vi "ReadData6.vi"() -> ()   [LabVIEW 2013]
uses:
  <vilib>/Utility/file.llb/Read From Spreadsheet File (DBL).vi
  <vilib>/Analysis/NI_AALPro.lvlib
  <vilib>/Analysis/NI_AALBase.lvlib
panel:
  out "Residual (V)":dbl=0.00030684756196116164 format="%#_3g"
  in  "1st sweep":i32=400
  in  "# of sweeps":i32=500
  out "Mean Error":dbl=0.0011249589574806795 format="%#_2g"
  out "Mean Area":dbl=0.018285831544207886 format="%#_4g"
  out "Spectrum #":i32=499
  out "Chars":i32=640716
  out "Fcen":dbl=213.0 format="%#_13g"
  in  "Fmin":dbl=212.8 format="%#_13g"
  in  "Fmax":dbl=213.2 format="%#_13g"
  out "# Data points":i32=81
  out "Peak Area (V-MHz)":dbl=0.016394272964669283 format="%#_3g"
  in  "Offset V":dbl=0.118 format="%#_3g"
  out "RMS Fit Error (V)":dbl=0.005928071319865591 format="%#_2g"
  in  "Start sigma (V)":dbl=0.01 format="%#_13g"
  in  "Start offset (V)":dbl format="%#_13g"
  out "FWHM (MHz)":dbl=0.06506841897793307 format="%#_3g"
  out "Center Freq (MHz)":dbl=213.0058317158631
  out "Amplitude (V)":dbl=0.2362707434086921 format="%#_3g"
  out "NMR Graph + Fit":cluster{cluster{dbl, "Numeric":dbl}[]}[](graph)=[{[{212.8, "Numeric"=2.363778842495368e-13}, {212.805, "Numeric"=8.902600611203184e-13}, {212.81, "Numeric"=3.2453766315993214e-12}, {212.815, "Numeric"=1.1451212757939673e-11}, {212.82000000000002, "Numeric"=3.910893842297015e-11}, {212.82500000000002, "Numeric"=1.2928220069997044e-10}, {212.83, "Numeric"=4.136562682898891e-10}, {212.835, "Numeric"=1.2810870705016114e-09}, {212.84, "Numeric"=3.8402177546863156e-09}, {212.845, "Numeric"=1.1142206913060541e-08}, {212.85000000000002, "Numeric"=3.129138254036874e-08}, {212.85500000000002, "Numeric"=8.505825122671001e-08}, {212.86, "Numeric"=2.237929040306476e-07}, {212.865, "Numeric"=5.699205791883683e-07}, {212.87, "Numeric"=1.4048195137059482e-06}, {212.875, "Numeric"=3.3516980604120123e-06}, {212.88, "Numeric"=7.740114936173332e-06}, {212.88500000000002, "Numeric"=1.7300876112483814e-05}, {212.89000000000001, "Numeric"=3.7430613688616755e-05}, {212.895, "Numeric"=7.838337581506647e-05}, {212.9, "Numeric"=0.00015887631007146483}, {212.905, "Numeric"=0.00031169690538213084}, {212.91, "Numeric"=0.0005918940865861797}, {212.915, "Numeric"=0.0010879117729213964}, {212.92000000000002, "Numeric"=0.0019354480411383043}, {212.925, "Numeric"=0.0033327867181186036}, {212.93, "Numeric"=0.005554841759608194}, {212.935, "Numeric"=0.008961362106463306}, {212.94, "Numeric"=0.013993118951798314}, {212.945, "Numeric"=0.021149163288258232}, {212.95, "Numeric"=0.030939266937258292}, {212.955, "Numeric"=0.04380916881708956}, {212.96, "Numeric"=0.06004241781343646}, {212.965, "Numeric"=0.07965068147769151}, {212.97, "Numeric"=0.10227252641250671}, {212.975, "Numeric"=0.12710617145852252}, {212.98, "Numeric"=0.1529017498753417}, {212.985, "Numeric"=0.17803133094838797}, {212.99, "Numeric"=0.2006404930271906}, {212.995, "Numeric"=0.21886630139748287}, {213.0, "Numeric"=0.23108799060021426}, {213.005, "Numeric"=0.23616417532011164}, {213.01, "Numeric"=0.23360859930023833}, {213.015, "Numeric"=0.22366694055030456}, {213.02, "Numeric"=0.20727786843888132}, {213.025, "Numeric"=0.18592690303473344}, {213.03, "Numeric"=0.16142459357518082}, {213.035, "Numeric"=0.13565485226578491}, {213.04, "Numeric"=0.11034156228151969}, {213.045, "Numeric"=0.08687225389622207}, {213.05, "Numeric"=0.06620049167290953}, {213.055, "Numeric"=0.048829188344330414}, {213.06, "Numeric"=0.034860688528937034}, {213.065, "Numeric"=0.0240896550155223}, {213.07, "Numeric"=0.01611251614068875}, {213.075, "Numeric"=0.010431201026979395}, {213.07999999999998, "Numeric"=0.006536472367332196}, {213.085, "Numeric"=0.003964520874143986}, {213.09, "Numeric"=0.002327427454472583}, {213.095, "Numeric"=0.0013225124280330355}, {213.1, "Numeric"=0.0007273803016944781}, {213.105, "Numeric"=0.0003872232932841738}, {213.10999999999999, "Numeric"=0.00019952603746162975}, {213.11499999999998, "Numeric"=9.951208960666663e-05}, {213.12, "Numeric"=4.8038593002941276e-05}, {213.125, "Numeric"=2.244620250801022e-05}, {213.13, "Numeric"=1.0151579953305604e-05}, {213.135, "Numeric"=4.443882496333521e-06}, {213.14, "Numeric"=1.8829104219250282e-06}, {213.14499999999998, "Numeric"=7.722091021339781e-07}, {213.14999999999998, "Numeric"=3.0653377834327045e-07}, {213.155, "Numeric"=1.1777684740226682e-07}, {213.16, "Numeric"=4.380056137615701e-08}, {213.165, "Numeric"=1.5766583426547003e-08}, {213.17, "Numeric"=5.493304516125009e-09}, {213.17499999999998, "Numeric"=1.85254139238475e-09}, {213.17999999999998, "Numeric"=6.047005050400953e-10}, {213.185, "Numeric"=1.9105170025266017e-10}, {213.19, "Numeric"=5.842512463679149e-11}, {213.195, "Numeric"=1.7293645527105895e-11}, {213.2, "Numeric"=4.954634507187724e-12}]}, {[{212.8, "Numeric"=0.004967440902254871}, {212.805, "Numeric"=-0.000296310531098675}, {212.81, "Numeric"=0.0010636834632183044}, {212.815, "Numeric"=0.00015015557407134416}, {212.82000000000002, "Numeric"=-0.003892310112972727}, {212.82500000000002, "Numeric"=-0.0014725852316157077}, {212.83, "Numeric"=-0.0023240371022075646}, {212.835, "Numeric"=-0.0017785572758793513}, {212.84, "Numeric"=-0.0022748424462961697}, {212.845, "Numeric"=7.121507719683851e-05}, {212.85000000000002, "Numeric"=-0.0002230889786892259}, {212.85500000000002, "Numeric"=0.00032456477231700603}, {212.86, "Numeric"=0.0013406520267375912}, {212.865, "Numeric"=0.002099375696453364}, {212.87, "Numeric"=0.0017847176492894966}, {212.875, "Numeric"=0.002550001113168818}, {212.88, "Numeric"=0.004441810296443963}, {212.88500000000002, "Numeric"=0.0011790998212828441}, {212.89000000000001, "Numeric"=0.005336953465366208}, {212.895, "Numeric"=0.005338041130925775}, {212.9, "Numeric"=0.004725033919440696}, {212.905, "Numeric"=0.005706776114412319}, {212.91, "Numeric"=0.006424525086713882}, {212.915, "Numeric"=0.007215254766544911}, {212.92000000000002, "Numeric"=0.004857810252633505}, {212.925, "Numeric"=0.007289539069902403}, {212.93, "Numeric"=0.002345657327556934}, {212.935, "Numeric"=0.004036724358499058}, {212.94, "Numeric"=-0.0006079531606907433}, {212.945, "Numeric"=-0.0028473223096827822}, {212.95, "Numeric"=-0.006544833228898432}, {212.955, "Numeric"=-0.008340857293439667}, {212.96, "Numeric"=-0.007216929546337303}, {212.965, "Numeric"=-0.004868895325288948}, {212.97, "Numeric"=0.003928908530641085}, {212.975, "Numeric"=0.008001653945618654}, {212.98, "Numeric"=0.012537203961757202}, {212.985, "Numeric"=0.01153786978325408}, {212.99, "Numeric"=0.006982401156061391}, {212.995, "Numeric"=0.0028520337900996987}, {213.0, "Numeric"=-0.0014723593376892111}, {213.005, "Numeric"=0.00010656764861838731}, {213.01, "Numeric"=-0.001386202902327774}, {213.015, "Numeric"=0.0048242795597373545}, {213.02, "Numeric"=0.009357326020612403}, {213.025, "Numeric"=0.01427539180160631}, {213.03, "Numeric"=0.01630984322515823}, {213.035, "Numeric"=0.012107750359368095}, {213.04, "Numeric"=0.007440163880240178}, {213.045, "Numeric"=-0.0030114071032364916}, {213.05, "Numeric"=-0.0064734824955001696}, {213.055, "Numeric"=-0.012187842950161915}, {213.06, "Numeric"=-0.01173342947034581}, {213.065, "Numeric"=-0.012007881761045145}, {213.07, "Numeric"=-0.010099588374144507}, {213.075, "Numeric"=-0.007674067897161301}, {213.07999999999998, "Numeric"=-0.008394259719215159}, {213.085, "Numeric"=-0.0052108737863584675}, {213.09, "Numeric"=-0.007589538010539377}, {213.095, "Numeric"=-0.005782368213358102}, {213.1, "Numeric"=-0.006088845641424775}, {213.105, "Numeric"=-0.0056869143330867886}, {213.10999999999999, "Numeric"=-0.00460497224075844}, {213.11499999999998, "Numeric"=-0.004840702366151415}, {213.12, "Numeric"=-0.0023242423109984802}, {213.125, "Numeric"=-0.0046342158474045785}, {213.13, "Numeric"=-0.0028768351709986197}, {213.135, "Numeric"=-0.002149579880285491}, {213.14, "Numeric"=0.00012217112966355715}, {213.14499999999998, "Numeric"=0.0004808905855907135}, {213.14999999999998, "Numeric"=0.0004397852216782692}, {213.155, "Numeric"=0.002021341374489691}, {213.16, "Numeric"=0.00179984490571965}, {213.165, "Numeric"=0.002898880909576887}, {213.17, "Numeric"=0.0015827486301250456}, {213.17499999999998, "Numeric"=0.003769076235776016}, {213.17999999999998, "Numeric"=0.0020295840182770275}, {213.185, "Numeric"=0.0004289023396565735}, {213.19, "Numeric"=0.0002501441304236038}, {213.195, "Numeric"=-0.0020244309700458182}, {213.2, "Numeric"=-0.003536579183989867}]}, {[{212.8, "Numeric"=0.004967440902491249}, {212.805, "Numeric"=-0.0002963105302084149}, {212.81, "Numeric"=0.001063683466463681}, {212.815, "Numeric"=0.00015015558552255691}, {212.82000000000002, "Numeric"=-0.0038923100738637887}, {212.82500000000002, "Numeric"=-0.0014725851023335071}, {212.83, "Numeric"=-0.002324036688551296}, {212.835, "Numeric"=-0.0017785559947922807}, {212.84, "Numeric"=-0.0022748386060784153}, {212.845, "Numeric"=7.122621940375157e-05}, {212.85000000000002, "Numeric"=-0.00022305768730668553}, {212.85500000000002, "Numeric"=0.0003246498305682327}, {212.86, "Numeric"=0.0013408758196416218}, {212.865, "Numeric"=0.002099945617032552}, {212.87, "Numeric"=0.0017861224688032027}, {212.875, "Numeric"=0.00255335281122923}, {212.88, "Numeric"=0.004449550411380137}, {212.88500000000002, "Numeric"=0.0011964006973953277}, {212.89000000000001, "Numeric"=0.0053743840790548255}, {212.895, "Numeric"=0.0054164245067408415}, {212.9, "Numeric"=0.004883910229512162}, {212.905, "Numeric"=0.006018473019794451}, {212.91, "Numeric"=0.007016419173300062}, {212.915, "Numeric"=0.008303166539466307}, {212.92000000000002, "Numeric"=0.00679325829377181}, {212.925, "Numeric"=0.010622325788021006}, {212.93, "Numeric"=0.007900499087165128}, {212.935, "Numeric"=0.012998086464962363}, {212.94, "Numeric"=0.013385165791107571}, {212.945, "Numeric"=0.01830184097857545}, {212.95, "Numeric"=0.02439443370835986}, {212.955, "Numeric"=0.03546831152364989}, {212.96, "Numeric"=0.05282548826709915}, {212.965, "Numeric"=0.07478178615240257}, {212.97, "Numeric"=0.1062014349431478}, {212.975, "Numeric"=0.13510782540414118}, {212.98, "Numeric"=0.1654389538370989}, {212.985, "Numeric"=0.18956920073164205}, {212.99, "Numeric"=0.20762289418325197}, {212.995, "Numeric"=0.22171833518758255}, {213.0, "Numeric"=0.22961563126252504}, {213.005, "Numeric"=0.23627074296873002}, {213.01, "Numeric"=0.23222239639791054}, {213.015, "Numeric"=0.22849122011004191}, {213.02, "Numeric"=0.21663519445949372}, {213.025, "Numeric"=0.20020229483633978}, {213.03, "Numeric"=0.17773443680033904}, {213.035, "Numeric"=0.147762602625153}, {213.04, "Numeric"=0.11778172616175986}, {213.045, "Numeric"=0.08386084679298558}, {213.05, "Numeric"=0.05972700917740937}, {213.055, "Numeric"=0.0366413453941685}, {213.06, "Numeric"=0.023127259058591223}, {213.065, "Numeric"=0.012081773254477155}, {213.07, "Numeric"=0.006012927766544244}, {213.075, "Numeric"=0.002757133129818095}, {213.07999999999998, "Numeric"=-0.0018577873518829636}, {213.085, "Numeric"=-0.0012463529122144813}, {213.09, "Numeric"=-0.005262110556066795}, {213.095, "Numeric"=-0.004459855785325067}, {213.1, "Numeric"=-0.005361465339730297}, {213.105, "Numeric"=-0.005299691039802616}, {213.10999999999999, "Numeric"=-0.00440544620329681}, {213.11499999999998, "Numeric"=-0.004741190276544749}, {213.12, "Numeric"=-0.0022762037179955394}, {213.125, "Numeric"=-0.004611769644896568}, {213.13, "Numeric"=-0.002866683591045314}, {213.135, "Numeric"=-0.002145135997789158}, {213.14, "Numeric"=0.00012405404008548218}, {213.14499999999998, "Numeric"=0.0004816627946928475}, {213.14999999999998, "Numeric"=0.0004400917554566125}, {213.155, "Numeric"=0.0020214591513370932}, {213.16, "Numeric"=0.001799888706281026}, {213.165, "Numeric"=0.0028988966761603133}, {213.17, "Numeric"=0.001582754123429562}, {213.17499999999998, "Numeric"=0.0037690780883174084}, {213.17999999999998, "Numeric"=0.002029584622977533}, {213.185, "Numeric"=0.0004289025307082737}, {213.19, "Numeric"=0.0002501441888487284}, {213.195, "Numeric"=-0.002024430952752173}, {213.2, "Numeric"=-0.0035365791790352326}]}]
  out "File size (bytes)":i32=1284000
  out "File name":string="C:\\Documents and Settings\\Patrick McGaughey\\Desktop\\rssmt\\NMR3489061581.xls"
  # "Gaussian Fit Results"
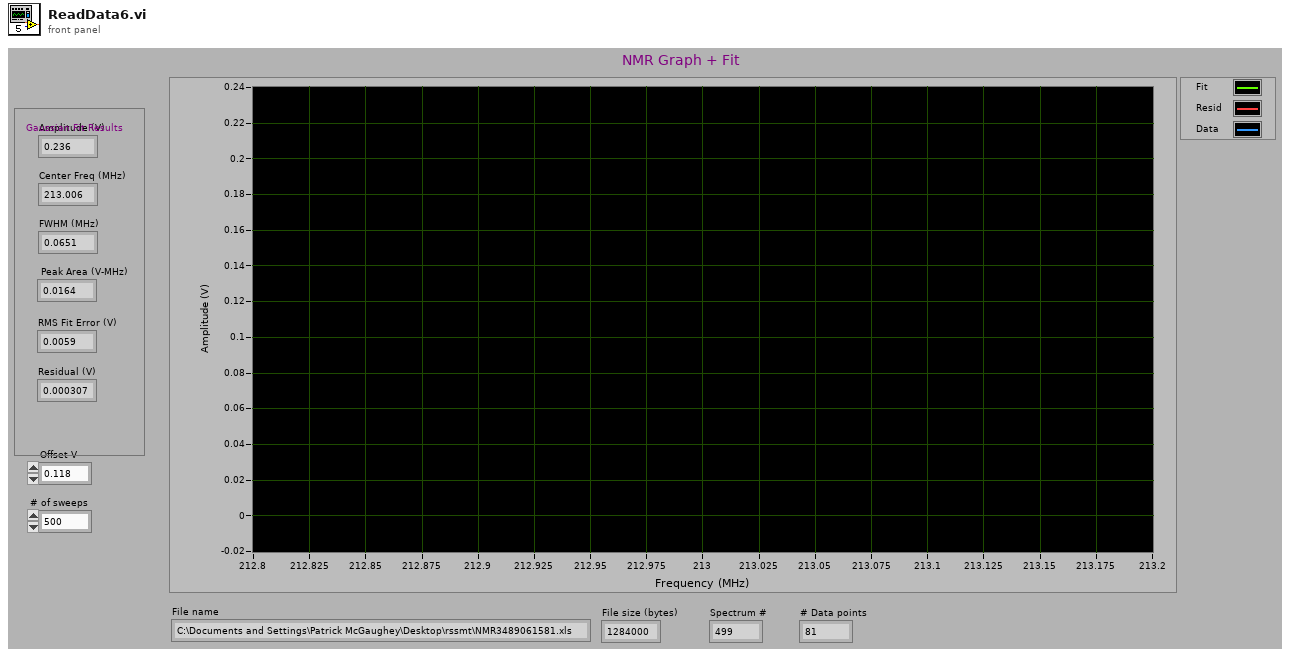
[diagram p1: front panel]
types:
  T1 = cluster{dbl, dbl, "Start sigma (V)":dbl, "Start offset (V)":dbl}
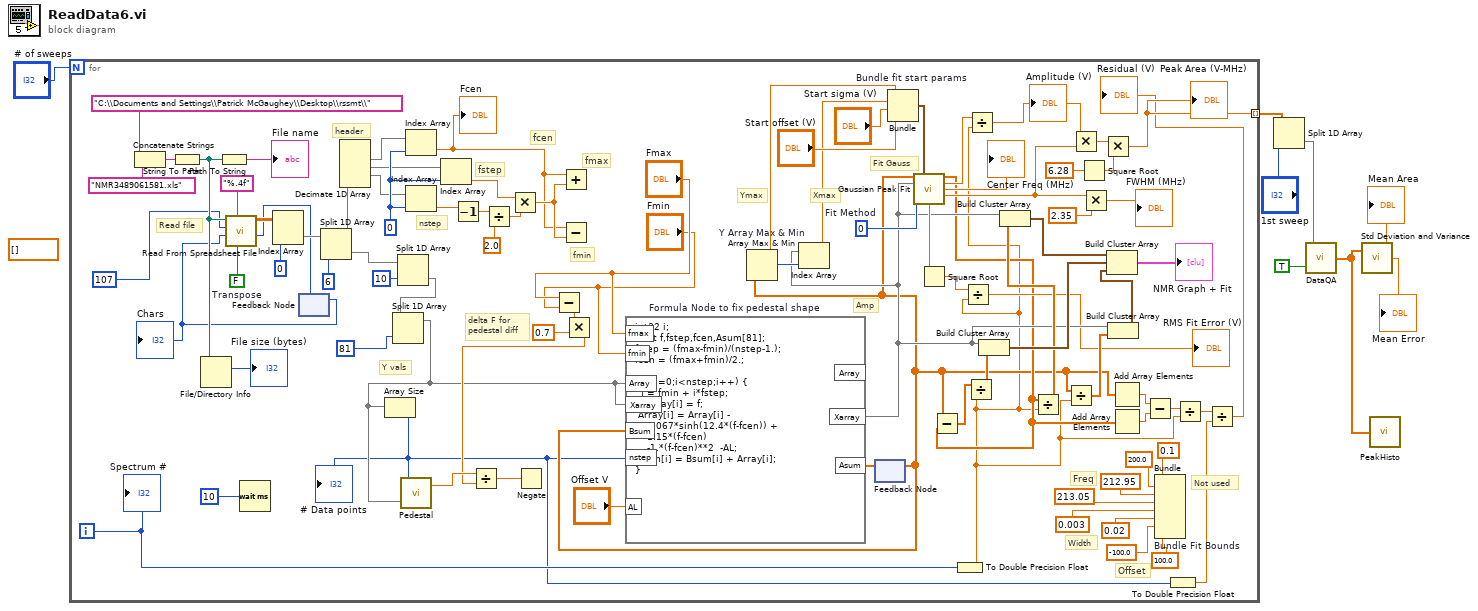
[diagram p0: block diagram]
diagram:
  (unwired) dbl[] []
  n1 = for {
    N: "# of sweeps" -> [_]
    tunnel: [w49] -> w3 mode=indexing
    i -> [w44]
    w60 = 0
    w86 = 0  # Fit Method
    w94 = FALSE  # Transpose
    # "Offset"
    # "Width"
    # "Freq"
    # "Not used"
    # "Fit Gauss"
    # "Read file"
    # "header"
    # "nstep"
    # "fstep"
    # "fcen"
    # "fmin"
    # "fmax"
    # "Amp"
    # "delta F for\npedestal diff"
    # "Ymax"
    # "Xmax"
    # "Y vals"
    n2 = Concatenate Strings "Concatenate Strings"("C:\\Documents and Settings\\Patrick McGaughey\\Desktop\\rssmt\\", "NMR3489061581.xls") -> (w97:string)
    n3 = String To Path(string=w97) -> (path=w93:path)
    n4 = File/Directory Info(path=w93) -> (size=→"File size (bytes)":i64)  [unwired: 1 in, 6 out]
    n5 = Path To String(path=w93) -> (string=→"File name":string)
    n6 = Wait (ms)(milliseconds to wait=10) -> ()  [unwired: 1 out]
    n7 = feedback #1() -> (w50:i32)  [unwired: 1 in]
    "Chars" <- w50
    n8 = call-poly <vilib>:"Read From Spreadsheet File.vi"("transpose (no:F)"=w94, "format (%.3f)"="%.4f", "start of read offset (chars.:0)"=w50, "number of rows (all:-1)"=107, "file path (dialog if empty)"=w93) -> ("mark after read (chars.)"=w51:i32, "all rows"=w68:dbl[][])  [unwired: 2 in, 3 out]
    n9 = Index Array "Index Array"(array=w68, index (col)=0) -> (element=w66:dbl[])  [unwired: 1 in]
    n10 = feedback-in #1(w51) -> ()
    n11 = Split 1D Array(array=w66, index=6) -> (first subarray=w69:dbl[], second subarray=w43:dbl[])
    n12 = Decimate 1D Array(w69) -> (w61:dbl[], w59:dbl[], w58:dbl[])  [unwired: 3 out]
    n13 = Split 1D Array(array=w43, index=10) -> (second subarray=w41:dbl[])  [unwired: 1 out]
    n14 = Split 1D Array(array=w41, index=81) -> (first subarray=w39:dbl[])  [unwired: 1 out]
    n15 = Array Size(array=w39) -> (size(s)=w10:i32)
    "# Data points" <- w10
    n16 = call "Pedestal.vi"("Varray"=w39, "ArraySize"=w10) -> ("L-R"=w80:dbl)  [unwired: 1 out]
    n17 = Index Array "Index Array"(array=w61, index=w60) -> (element=w52:dbl)
    "Fcen" <- w52
    n18 = Index Array(array=w58, index=w60) -> (element=w56:dbl)
    n19 = Index Array(array=w59, index=w60) -> (element=w57:dbl)
    n20 = Decrement(x=w56) -> (x-1=w65:dbl)
    n21 = Divide(x=w65, y=2.0) -> (x/y=w63:dbl)
    n22 = Multiply(x=w57, y=w63) -> (x*y=w62:dbl)
    n23 = Subtract(x="Fmax", y="Fmin") -> (x-y=w78:dbl)
    n24 = Add(x=w52, y=w62) -> ()  [unwired: 1 out]
    n25 = Subtract(x=w52, y=w62) -> ()  [unwired: 1 out]
    n26 = Multiply(x=w78, y=0.7) -> (x*y=w77:dbl)
    n27 = Divide(x=w80, y=w77) -> (x/y=w76:dbl)
    n28 = Negate(x=w76) -> ()  [unwired: 1 out]
    n29 = feedback #2() -> (w17:dbl[])  [unwired: 1 in]
    n30 = formula code="int32 i;\nfloat f,fstep,fcen,Asum[81];\nfstep = (fmax-fmin)/(nstep-1.);\nfcen = (fmax+fmin)/2.;\n\nfor (i=0;i<nstep;i++) {\n  f = fmin + i*fstep;\n  Xarray[i] = f;\n Array[i] = Array[i] - \n    0.067*sinh(12.4*(f-fcen)) +\n    1.15*(f-fcen)  \n    -1.*(f-fcen)**2  -AL;\nAsum[i] = Bsum[i] + Array[i];\n}" "Formula Node to fix pedestal shape"("nstep"=w10, "fmin"="Fmin", "fmax"="Fmax", "AL"="Offset V", "Array"=w39, "Xarray"=w39, "Bsum"=w17) -> ("Xarray"=w32:dbl[], "Asum"=w48:dbl[])  [unwired: 1 out]
    n31 = Array Max & Min "Y Array Max & Min"(array=w17) -> (max value=w85:dbl, max index (indices)=w84:i32)  [unwired: 2 out]
    n32 = Index Array "Index Array"(array=w32, index=w84) -> (element=w74:dbl)
    n33 = feedback-in #2(w48) -> ()
    n34 = Bundle "Bundle fit start params"(w85, w74, "Start sigma (V)"="Start sigma (V)", "Start offset (V)"="Start offset (V)") -> (w89:T1)  [unwired: 1 in]
    n35 = call <vilib>:"Gaussian Peak Fit.vi"("Y"=w17, "initial guess"=w89, "X"=w32, "method"=w86) -> ("Best Gaussian Fit"=w18:dbl[], "amplitude"=w34:dbl, "center"=→"Center Freq (MHz)":dbl, "standard deviation"=w73:dbl, "residue"=w75:dbl)  [unwired: 5 in, 2 out]
    n36 = Square Root(x=w75) -> (sqrt(x)=w29:dbl)
    n37 = Subtract(x=w17, y=w18) -> (x-y=w46:dbl[])
    n38 = To Double Precision Float(number=w44) -> (double precision float=w13:dbl)
    n39 = Divide(x=w29, y=w13) -> (x/y=→"RMS Fit Error (V)":dbl)
    n40 = Divide(x=w46, y=w13) -> (x/y=w45:dbl[])
    n41 = Divide(x=w34, y=w13) -> (x/y=w33:dbl)
    "Amplitude (V)" <- w33
    n42 = Build Cluster Array ("Index & Bundle Cluster Array")(w32, w45) -> (w47:cluster{dbl, dbl}[])
    n43 = Divide(x=w18, y=w13) -> (x/y=w35:dbl[])
    n44 = Build Cluster Array ("Index & Bundle Cluster Array")(w32, w35) -> (w55:cluster{dbl, dbl}[])
    n45 = Divide(x=w17, y=w13) -> (x/y=w30:dbl[])
    n46 = Multiply(x=w33, y=w73) -> (x*y=w81:dbl)
    n47 = Square Root(x=6.28) -> (sqrt(x)=w82:dbl)
    n48 = Multiply(x=w73, y=2.35) -> (x*y=→"FWHM (MHz)":dbl)
    n49 = Multiply(x=w81, y=w82) -> (x*y=w49:dbl)
    "Peak Area (V-MHz)" <- w49
    n50 = Build Cluster Array ("Index & Bundle Cluster Array")(w32, w30) -> (w31:cluster{dbl, dbl}[])
    n51 = Build Cluster Array "Build Cluster Array"(w55, w47, w31) -> (→"NMR Graph + Fit":cluster{cluster{dbl, dbl}[]}[])
    n52 = Add Array Elements(numeric array=w17) -> (sum=w15:dbl)
    n53 = Add Array Elements(numeric array=w18) -> (sum=w16:dbl)
    n54 = Subtract(x=w15, y=w16) -> (x-y=w14:dbl)
    n55 = Bundle "Bundle Fit Bounds"(0.1, 200.0, 212.95, 213.05, 0.003, 0.02, -100.0, 100.0) -> ()  [unwired: 1 in, 1 out]
    n56 = To Double Precision Float(number=w10) -> (double precision float=w9:dbl)
    n57 = Divide(x=w14, y=w13) -> (x/y=w12:dbl)
    n58 = Divide(x=w12, y=w9) -> (x/y=→"Residual (V)":dbl)
    "Spectrum #" <- w44
  }
  n59 = Split 1D Array(array=w3, index="1st sweep") -> (second subarray=w1:dbl[])  [unwired: 1 out]
  n60 = call "DataQA.vi"("Quality cuts"=TRUE, "Data In"=w1) -> ("Data Out"=w4:dbl[])
  n61 = call <vilib>:"Std Deviation and Variance.vi"("X"=w4) -> ("mean"=→"Mean Area":dbl, "standard deviation"=→"Mean Error":dbl)  [unwired: 1 in, 1 out]
  n62 = call "PeakHisto.vi"("Data Out"=w4) -> ()  [unwired: 1 out]
